vi "SearchMatch.vi"(8 "Error In":errorcluster, 11 "data_from2d3d":i32[](array[numeric])) -> (0 "Error Out":errorcluster, 1 "Elements Selected":string[][](table), 3 "data out":T2, 4 "Param Calibrazione":T1, 5 "List ROI out":dbl[][](array[numeric]))   [LabVIEW 2023]
uses:
  control/param_calibrazione.ctl
  <vilib>/Analysis/1siggen.llb/Ramp Pattern by Samples.vi
  control/global name path.vi
  queue/Front Panel Message Queue.lvlib
  <vilib>/Analysis/NI_AALBase.lvlib
panel:
  out "Saving Parth":path
  in  "name sample":bool
  in  "concentration":bool
  in  "Load Calibration":path
  out "name":string
  in  "Save":bool
  out "XY Graph":T2(graph)
  in  "select":bool
  out "Peaks Found":string[][](table)
  in  "Search Peak":bool
  in  "width":i32=80 min=3
  in  "threshold":dbl=1500.0 format="%0.2f"
  out "Spectrum":cluster{"Channels":dbl[], "Intensity":dbl[]}[](graph)
  out "Data In":T3(graph)
  in  "load":bool
  in  "open":bool
  in  "calib":bool
  in  "Stop":bool
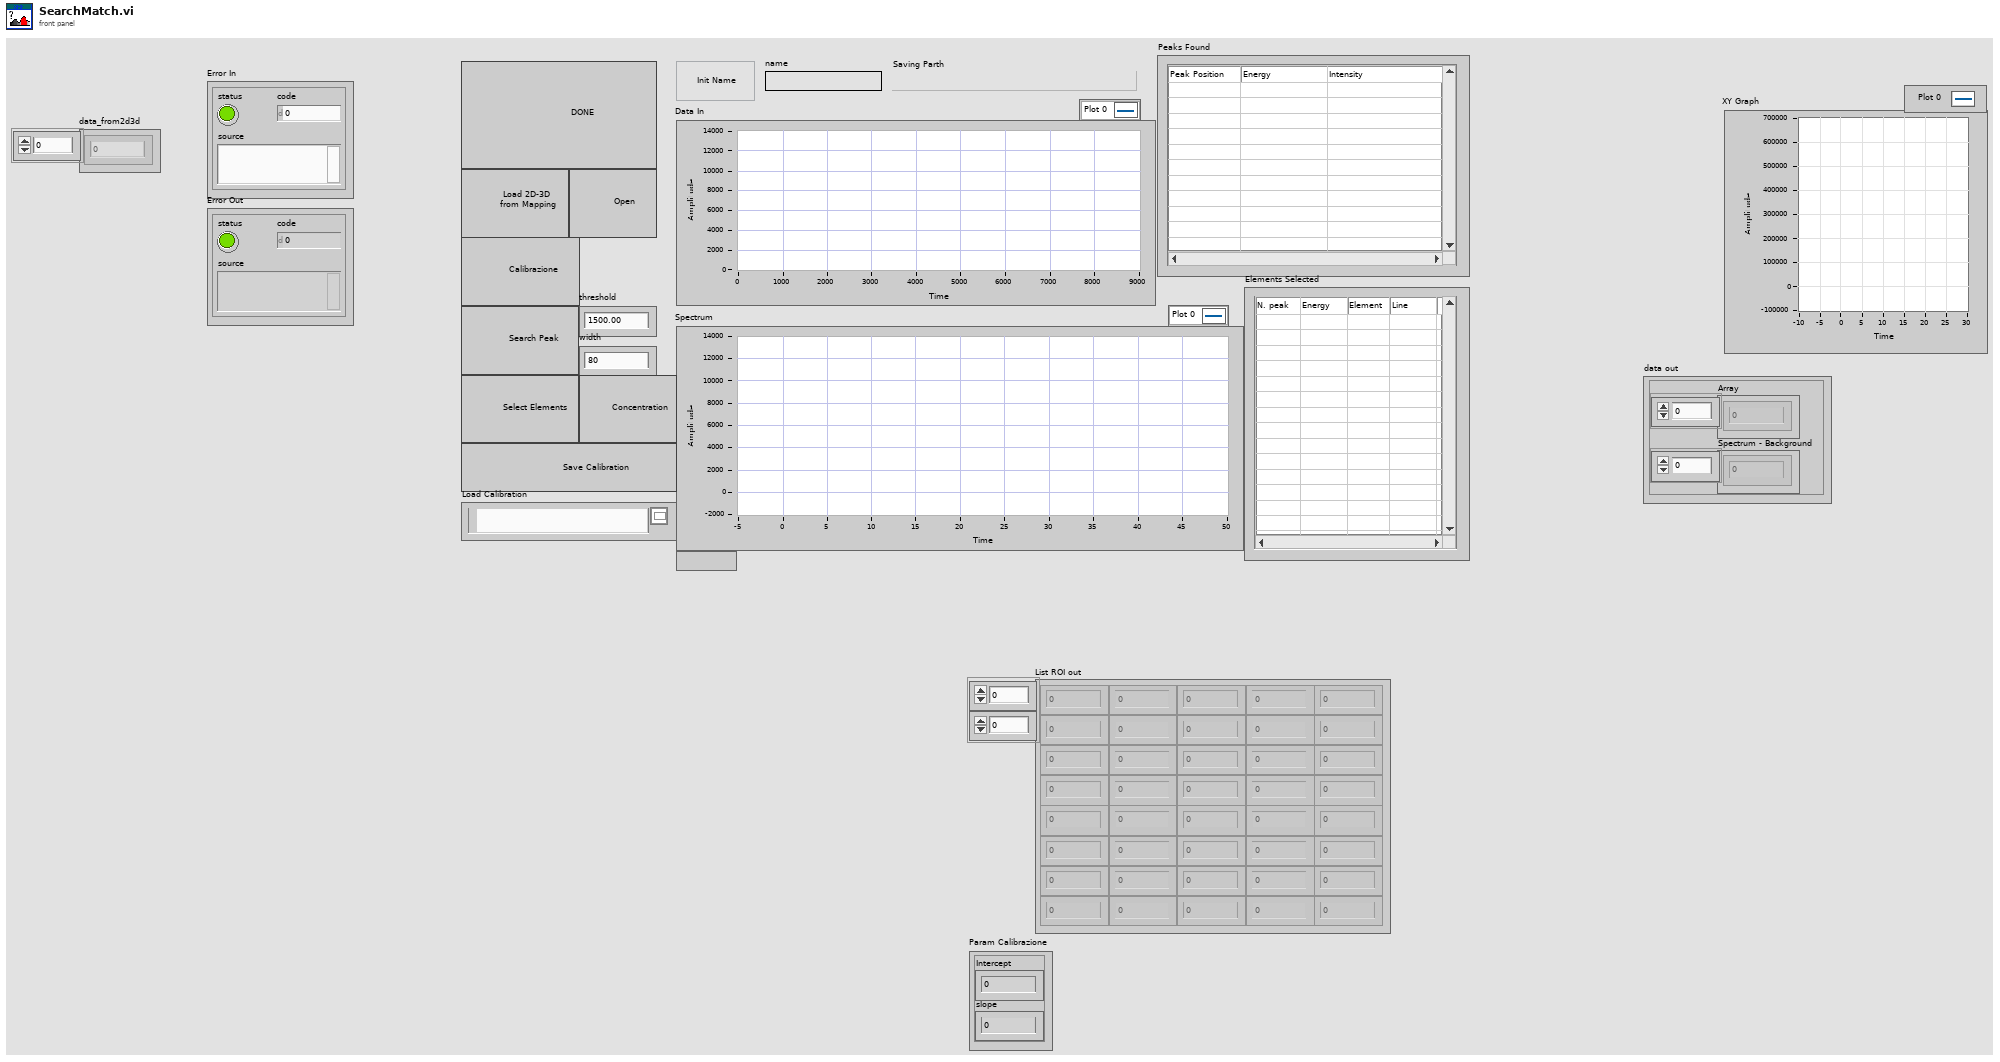
[diagram p1: front panel]
types:
  T1 = typedef "param_calibrazione.ctl" = cluster{"Intercept":dbl, "slope":dbl}
  T2 = cluster{"Array":dbl[], "Spectrum - Background":dbl[]}
  T3 = cluster{"Ramp Pattern":dbl[], "data_from2d3d":i32[]}
  T4 = typedef "Front Panel Message Queue.lvlib/Calibrazione Message Queues.ctl" = cluster{"Main":refnum<queue>, "Data":refnum<queue>}
  T5 = cluster{"Array":dbl[], "Spectrum - Background":dbl[]}[]
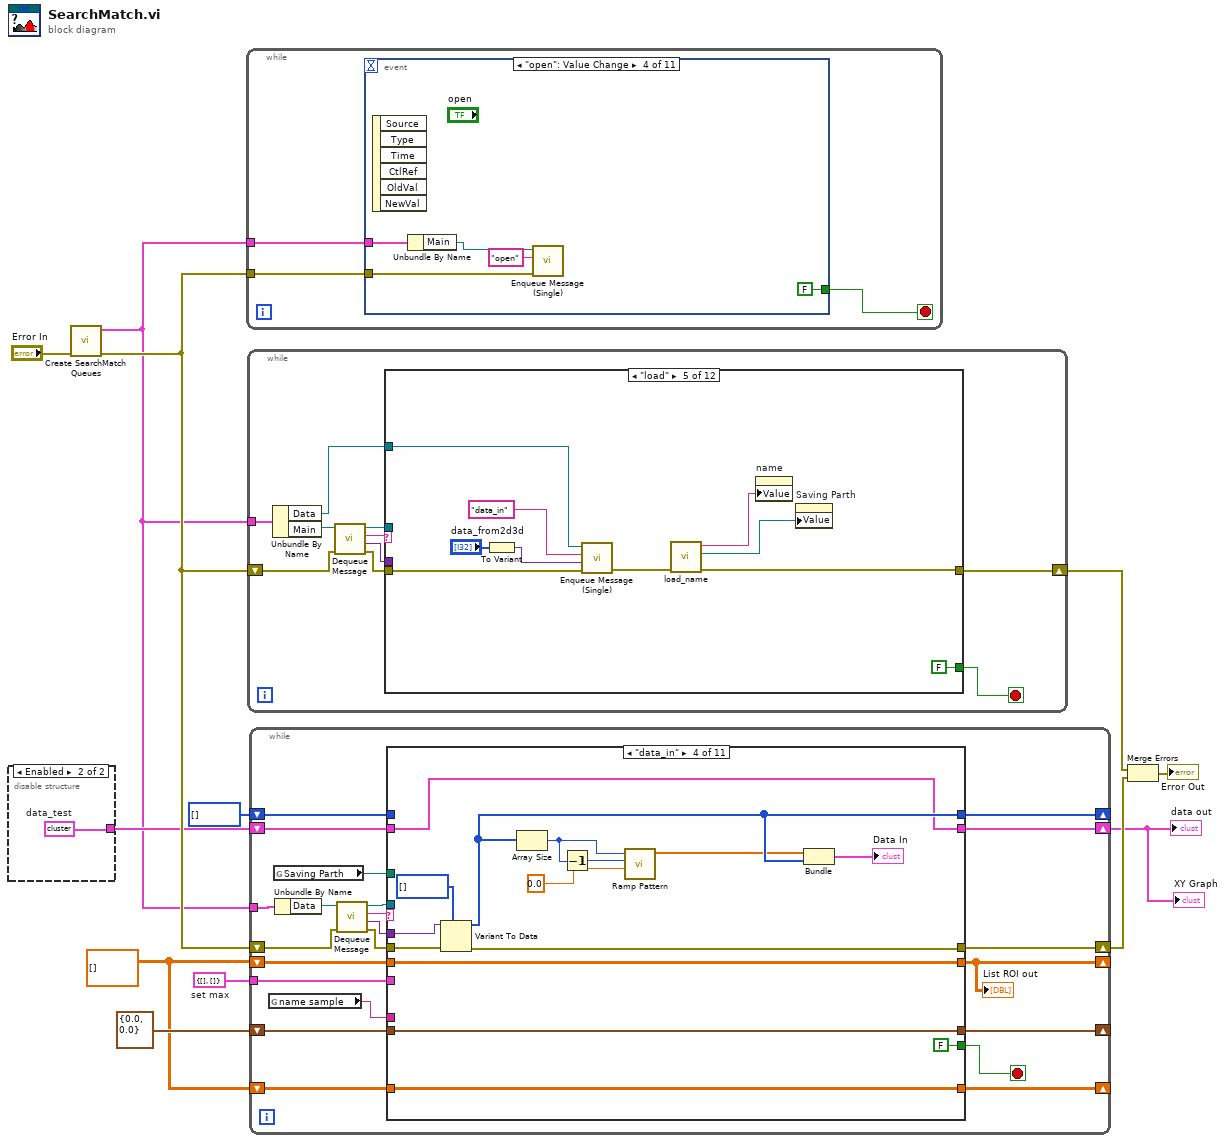
[diagram p0: block diagram]
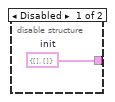
[diagram p2: hidden frame]
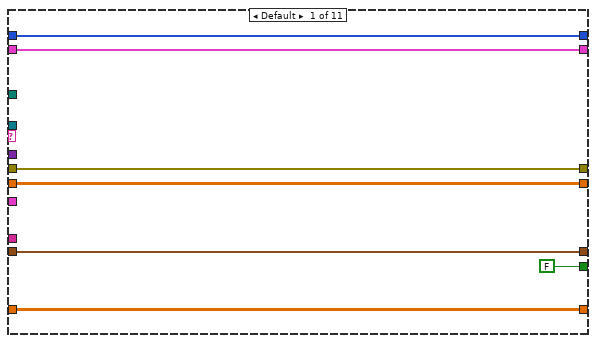
[diagram p3: hidden frame]
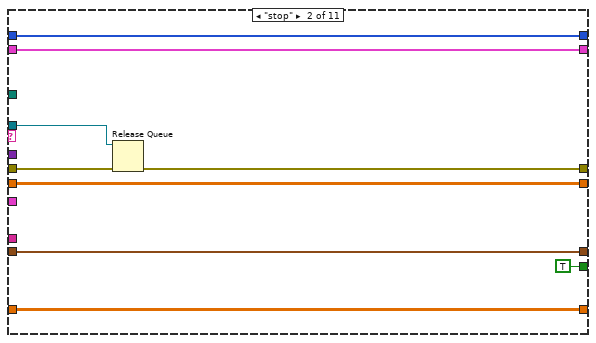
[diagram p4: hidden frame]
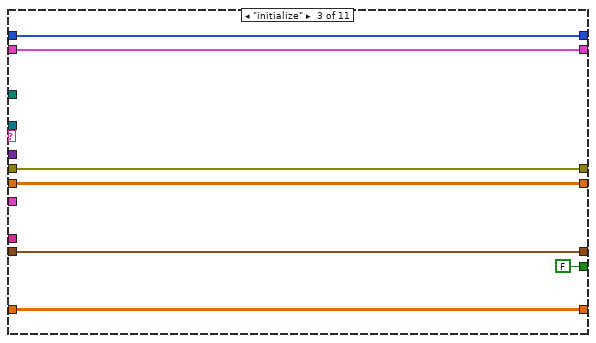
[diagram p5: hidden frame]
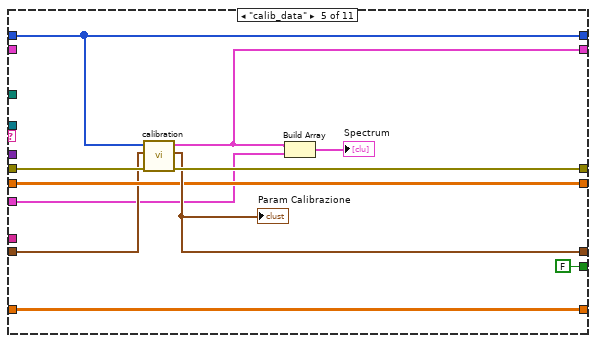
[diagram p6: hidden frame]
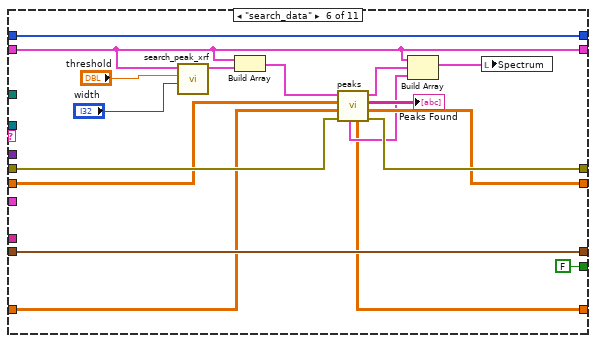
[diagram p7: hidden frame]
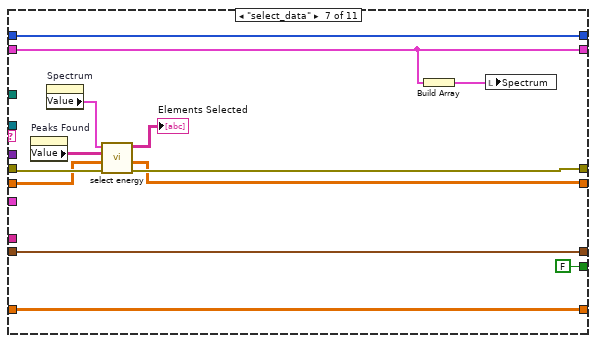
[diagram p8: hidden frame]
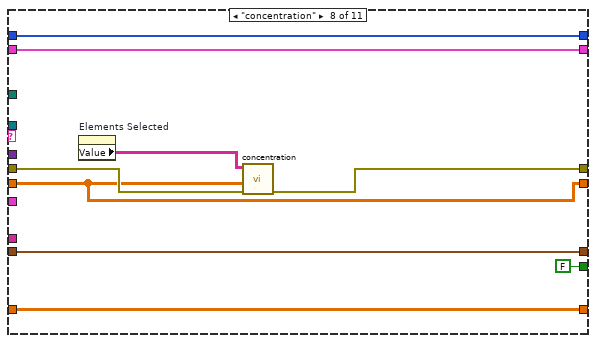
[diagram p9: hidden frame]
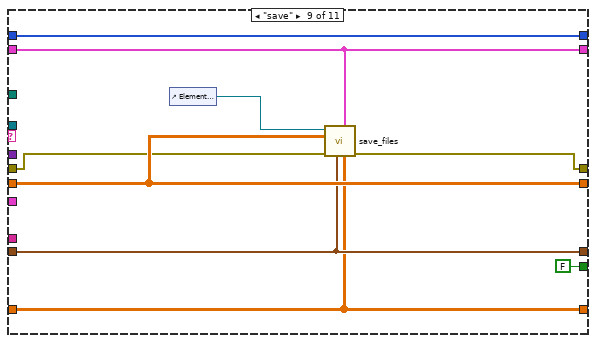
[diagram p10: hidden frame]
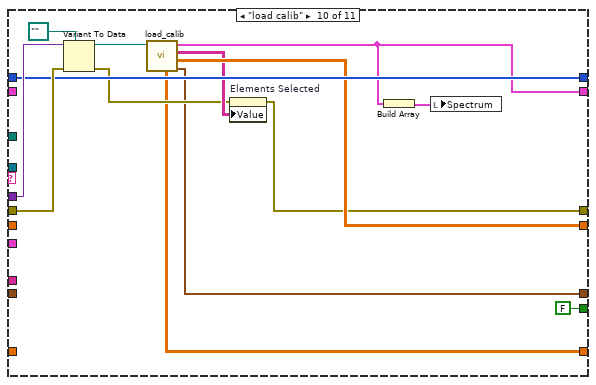
[diagram p11: hidden frame]
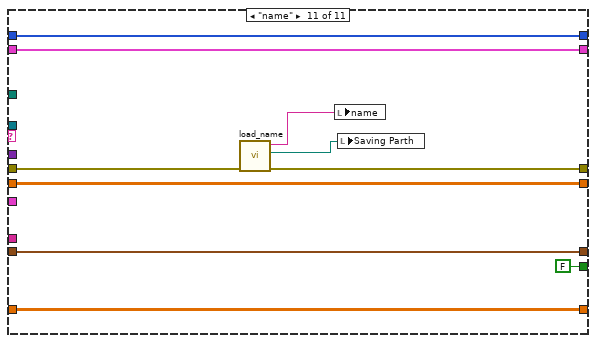
[diagram p12: hidden frame]
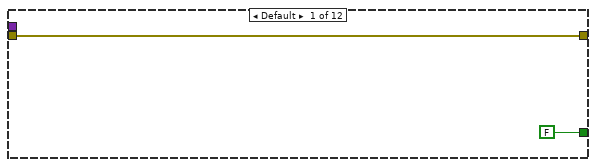
[diagram p13: hidden frame]
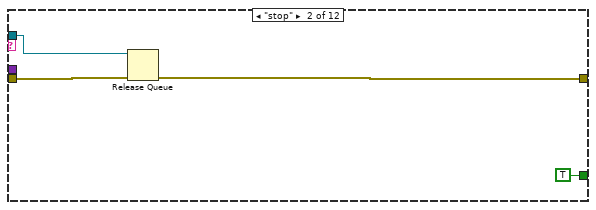
[diagram p14: hidden frame]
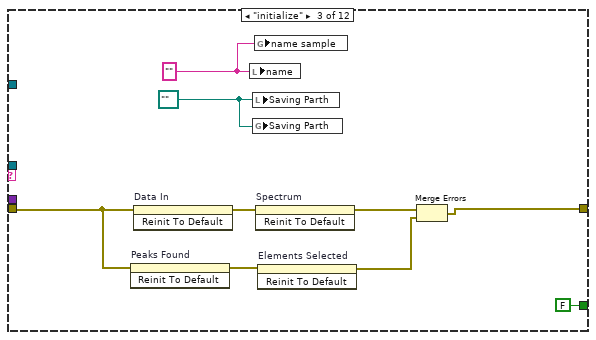
[diagram p15: hidden frame]
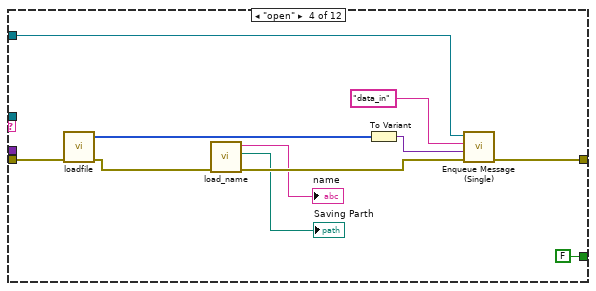
[diagram p16: hidden frame]
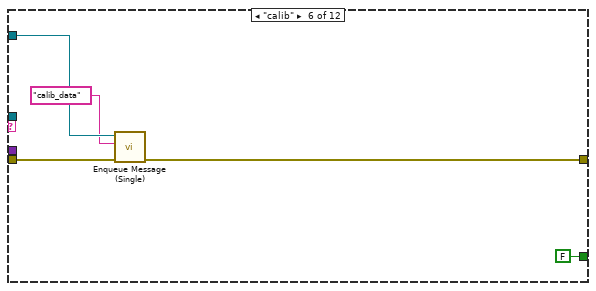
[diagram p17: hidden frame]
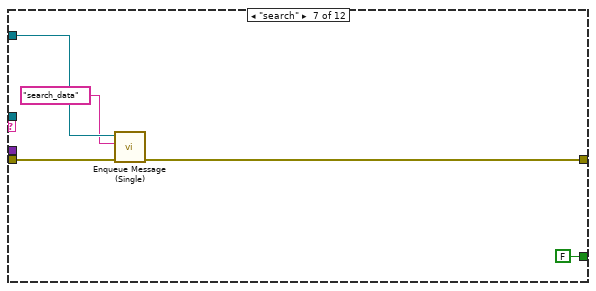
[diagram p18: hidden frame]
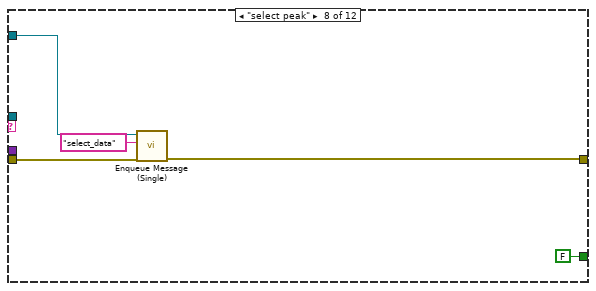
[diagram p19: hidden frame]
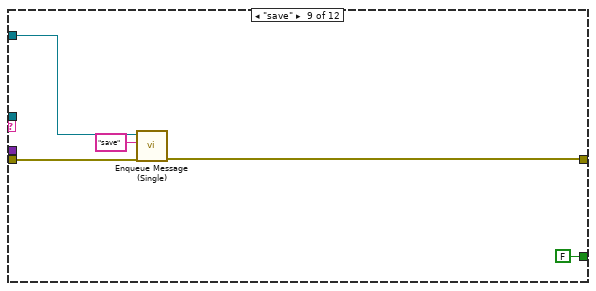
[diagram p20: hidden frame]
diagram:
  w1 = dbl[][] [] ("List ROI")
  w5 = cluster{"Channels":dbl[], "Intensity":dbl[]} {"Channels"=[], "Intensity"=[]}  # set max
  n1 = disable-structure shown="Enabled" {
    disable-tunnel: [w13 w14] -> w6
    frame Disabled {
      w13 = T2 {"Array"=[], "Spectrum - Background"=[]}  # init
    }
    frame Enabled {
      w14 = T2 {"Array"=array[8192 elements], "Spectrum - Background"=array[8192 elements]}  # data_test
    }
  }
  n2 = call "Create SearchMatch Queues.vi"("error in (no error)"="Error In") -> ("error out"=w9:errorcluster, "Message Queues"=w2:T4)  [unwired: 9 in]
  n3 = while {
    tunnel: w9 -> [w16]
    tunnel: w2 -> [w15]
    stop <- w17 stop-if-true
    n4 = event shown="[3] \"open\": Value Change" {
      selector: _ -> [_ _ _ _ _ _ _ _ _ _ _]
      dyn-events: _ -> [_ _ _ _ _ _ _ _ _ _ _]
      timeout: _ -> [_ _ _ _ _ _ _ _ _ _ _]
      tunnel: [FALSE TRUE FALSE FALSE FALSE FALSE FALSE FALSE FALSE FALSE FALSE] -> w17
      tunnel: w16 -> [_ w25 w30 w35 w41 w46 w49 w54 w61 w66 w72]
      tunnel: w15 -> [_ w24 w29 w34 w39 w44 w51 w56 w60 w65 w71]
      event Timeout {
        n5 = event-data() -> ()  [unwired: 1 in, 3 out]
      }
      event "Stop": Value Change {
        w22 = TRUE ("Priority Message? (F)")
        w21 = "stop" ("Message")
        n6 = event-data() -> ()  [unwired: 1 in, 6 out]
        n7 = Unbundle By Name(w24) -> ("Main"=w19:refnum<queue>, "Data"=w20:refnum<queue>)
        n8 = call "Enqueue Message (Single).vi"("Priority Message? (F)"=w22, "error in (no error)"=w25, "Message"=w21, "Message Queue"=w20) -> ("error out"=w23:errorcluster)  [unwired: 6 in, 1 out]
        n9 = call "Enqueue Message (Single).vi"("Priority Message? (F)"=w22, "error in (no error)"=w23, "Message"=w21, "Message Queue"=w19) -> ()  [unwired: 6 in, 2 out]
      }
      event "load": Value Change {
        n10 = event-data() -> ()  [unwired: 1 in, 6 out]
        n11 = Unbundle By Name(w29) -> ("Main"=w28:refnum<queue>)
        n12 = call "Enqueue Message (Single).vi"("error in (no error)"=w30, "Message"="load", "Message Queue"=w28) -> ()  [unwired: 7 in, 2 out]
      }
      event "open": Value Change {
        n13 = event-data() -> ()  [unwired: 1 in, 6 out]
        n14 = Unbundle By Name(w34) -> ("Main"=w33:refnum<queue>)
        n15 = call "Enqueue Message (Single).vi"("error in (no error)"=w35, "Message"="open", "Message Queue"=w33) -> ()  [unwired: 7 in, 2 out]
      }
      event "calib": Value Change {
        n16 = event-data() -> ()  [unwired: 1 in, 6 out]
        n17 = Unbundle By Name(w39) -> ("Main"=w38:refnum<queue>)
        n18 = call "Enqueue Message (Single).vi"("error in (no error)"=w41, "Message"="calib", "Message Queue"=w38) -> ()  [unwired: 7 in, 2 out]
      }
      event "Search Peak": Value Change {
        n19 = event-data() -> ()  [unwired: 1 in, 6 out]
        n20 = Unbundle By Name(w44) -> ("Main"=w43:refnum<queue>)
        n21 = call "Enqueue Message (Single).vi"("error in (no error)"=w46, "Message"="search", "Message Queue"=w43) -> ()  [unwired: 7 in, 2 out]
      }
      event "select": Value Change {
        n22 = event-data() -> ()  [unwired: 1 in, 6 out]
        n23 = Unbundle By Name(w51) -> ("Main"=w50:refnum<queue>)
        n24 = call "Enqueue Message (Single).vi"("error in (no error)"=w49, "Message"="select peak", "Message Queue"=w50) -> ()  [unwired: 7 in, 2 out]
      }
      event "Save": Value Change {
        n25 = event-data() -> ()  [unwired: 1 in, 6 out]
        n26 = Unbundle By Name(w56) -> ("Main"=w55:refnum<queue>)
        n27 = call "Enqueue Message (Single).vi"("error in (no error)"=w54, "Message"="save", "Message Queue"=w55) -> ()  [unwired: 7 in, 2 out]
      }
      event "Load Calibration": Value Change {
        n28 = event-data() -> ()  [unwired: 1 in, 6 out]
        n29 = To Variant(anything="Load Calibration") -> (Variant=w58:variant)
        n30 = Unbundle By Name(w60) -> ("Main"=w63:refnum<queue>)
        n31 = call "Enqueue Message (Single).vi"("error in (no error)"=w61, "Message Data"=w58, "Message"="load calib", "Message Queue"=w63) -> ()  [unwired: 6 in, 2 out]
      }
      event "name sample": Value Change {
        n32 = event-data() -> ()  [unwired: 1 in, 6 out]
        n33 = Unbundle By Name(w65) -> ("Main"=w68:refnum<queue>)
        n34 = call "Enqueue Message (Single).vi"("error in (no error)"=w66, "Message"="name", "Message Queue"=w68) -> ()  [unwired: 7 in, 2 out]
      }
      event "concentration": Value Change {
        n35 = event-data() -> ()  [unwired: 1 in, 6 out]
        n36 = Unbundle By Name(w71) -> ("Main"=w70:refnum<queue>)
        n37 = call "Enqueue Message (Single).vi"("error in (no error)"=w72, "Message"="concentration", "Message Queue"=w70) -> ()  [unwired: 7 in, 2 out]
      }
    }
  }
  n38 = while {
    shift-right: [w79] -> w10
    shift-left: w9 -> [w83]
    tunnel: w2 -> [w74]
    stop <- w81 stop-if-true
    n39 = Unbundle By Name(w74) -> ("Data"=w76:refnum<queue>, "Main"=w78:refnum<queue>)
    n40 = call "Dequeue Message.vi"("error in (no error)"=w83, "Message Queue"=w78) -> ("error out"=w80:errorcluster, "Message Data"=w75:variant, "Message"=w82:string, "dup Message Queue"=w77:refnum<queue>)  [unwired: 5 in, 1 out]
    n41 = case shown="\"load\"" w82 {
      tunnel: [FALSE TRUE FALSE FALSE FALSE FALSE FALSE FALSE FALSE FALSE FALSE FALSE] -> w81
      tunnel: w80 -> [w84 w88 w96 w108 w115 w123 w128 w134 w139 w145 w150 w154]
      tunnel: [w84 w87 w92 w103 w110 w122 w127 w132 w137 w143 w148 w152] -> w79
      tunnel: w77 -> [_ w86 _ _ _ _ _ _ _ _ _ _]
      tunnel: w76 -> [_ _ _ w107 w118 w121 w126 w133 w138 w144 w149 w153]
      tunnel: w75 -> [_ _ _ _ _ _ _ _ _ w140 _ _]
      frame Default {
      }
      frame "stop" {
        n42 = Release Queue(queue=w86, error in (no error)=w88) -> (error out=w87:errorcluster)  [unwired: 1 in, 2 out]
      }
      frame "initialize" {
        w91 = path ""
        w90 = ""
        n43 = invoke on="Peaks Found" class="Tbl (strict)" method="Reinit To Default"(error in=w96) -> (error out=w95:errorcluster)  [unwired: 2 in, 2 out]
        n44 = invoke on="Data In" class="XYGraph (strict)" method="Reinit To Default"(error in=w96) -> (error out=w97:errorcluster)  [unwired: 2 in, 2 out]
        n45 = local write "name"(w90) -> ()
        n46 = local write "Saving Parth"(w91) -> ()
        n47 = global write "global name path.vi" "Saving Parth"(w91) -> ()
        n48 = global write "global name path.vi" "name sample"(w90) -> ()
        n49 = invoke on="Spectrum" class="XYGraph (strict)" method="Reinit To Default"(error in=w97) -> (error out=w94:errorcluster)  [unwired: 2 in, 2 out]
        n50 = invoke on="Elements Selected" class="Tbl (strict)" method="Reinit To Default"(error in=w95) -> (error out=w93:errorcluster)  [unwired: 2 in, 2 out]
        n51 = Merge Errors(w94, w93) -> (w92:errorcluster)
      }
      frame "open" {
        n52 = call "loadfile.vi"("Error In"=w108) -> ("Error Out"=w102:errorcluster, "Data"=w106:i64[])  [unwired: 9 in]
        n53 = call "load_name.vi"("error in"=w102) -> ("error out"=w101:errorcluster, "Saving Path Out"=→"Saving Parth":path, "Name Out"=→"name":string)  [unwired: 8 in]
        n54 = To Variant(anything=w106) -> (Variant=w105:variant)
        n55 = call "Enqueue Message (Single).vi"("error in (no error)"=w101, "Message Data"=w105, "Message"="data_in", "Message Queue"=w107) -> ("error out"=w103:errorcluster)  [unwired: 6 in, 1 out]
      }
      frame "load" {
        n56 = To Variant(anything="data_from2d3d") -> (Variant=w117:variant)
        n57 = call "Enqueue Message (Single).vi"("error in (no error)"=w115, "Message Data"=w117, "Message"="data_in", "Message Queue"=w118) -> ("error out"=w111:errorcluster)  [unwired: 6 in, 1 out]
        n58 = call "load_name.vi"("error in"=w111) -> ("error out"=w110:errorcluster, "Saving Path Out"=w113:path, "Name Out"=w112:string)  [unwired: 8 in]
        n59 = property on="name" class="Str"("Value"=w112) -> ()  [unwired: 2 in, 2 out]
        n60 = property on="Saving Parth" class="Path"("Value"=w113) -> ()  [unwired: 2 in, 2 out]
      }
      frame "calib" {
        n61 = call "Enqueue Message (Single).vi"("error in (no error)"=w123, "Message"="calib_data", "Message Queue"=w121) -> ("error out"=w122:errorcluster)  [unwired: 7 in, 1 out]
      }
      frame "search" {
        n62 = call "Enqueue Message (Single).vi"("error in (no error)"=w128, "Message"="search_data", "Message Queue"=w126) -> ("error out"=w127:errorcluster)  [unwired: 7 in, 1 out]
      }
      frame "select peak" {
        n63 = call "Enqueue Message (Single).vi"("error in (no error)"=w134, "Message"="select_data", "Message Queue"=w133) -> ("error out"=w132:errorcluster)  [unwired: 7 in, 1 out]
      }
      frame "save" {
        n64 = call "Enqueue Message (Single).vi"("error in (no error)"=w139, "Message"="save", "Message Queue"=w138) -> ("error out"=w137:errorcluster)  [unwired: 7 in, 1 out]
      }
      frame "load calib" {
        n65 = call "Enqueue Message (Single).vi"("error in (no error)"=w145, "Message Data"=w140, "Message"="load calib", "Message Queue"=w144) -> ("error out"=w143:errorcluster)  [unwired: 6 in, 1 out]
      }
      frame "name" {
        n66 = call "Enqueue Message (Single).vi"("error in (no error)"=w150, "Message"="name", "Message Queue"=w149) -> ("error out"=w148:errorcluster)  [unwired: 7 in, 1 out]
      }
      frame "concentration" {
        n67 = call "Enqueue Message (Single).vi"("error in (no error)"=w154, "Message"="concentration", "Message Queue"=w153) -> ("error out"=w152:errorcluster)  [unwired: 7 in, 1 out]
      }
    }
  }
  n68 = while {
    shift-right: [w172] -> w8
    shift-left: w9 -> [w176]
    shift-right: [w169] -> _
    shift-left: i64[] [] ("data_from2d3d") -> [w168]
    shift-right: [w167] -> w3
    shift-left: w6 -> [w166]
    tunnel: w5 -> [w165]
    shift-right: [w164] -> _
    shift-left: T1 {"Intercept"=0.0, "slope"=0.0} ("Param Calibrazione") -> [w163]
    shift-right: [w162] -> _
    shift-left: w1 -> [w161]
    tunnel: w2 -> [w160]
    shift-right: [w159] -> _
    shift-left: w1 -> [w158]
    stop <- w174 stop-if-true
    n69 = global read "global name path.vi" "name sample"() -> (w156:string)
    n70 = global read "global name path.vi" "Saving Parth"() -> (w157:path)
    n71 = Unbundle By Name(w160) -> ("Data"=w177:refnum<queue>)
    n72 = call "Dequeue Message.vi"("error in (no error)"=w176, "Message Queue"=w177) -> ("error out"=w173:errorcluster, "Message Data"=w170:variant, "Message"=w175:string, "dup Message Queue"=w171:refnum<queue>)  [unwired: 5 in, 1 out]
    n73 = case shown="\"data_in\"" w175 {
      tunnel: [FALSE TRUE FALSE FALSE FALSE FALSE FALSE FALSE FALSE FALSE FALSE] -> w174
      tunnel: w173 -> [w183 w192 w199 w215 w225 w239 w255 w263 w269 w288 w293]
      tunnel: [w183 w190 w199 w212 w224 w238 w254 w262 w272 w280 w292] -> w172
      tunnel: w171 -> [_ w191 _ _ _ _ _ _ _ _ _]
      tunnel: w170 -> [_ _ _ w214 _ _ _ _ _ w287 _]
      tunnel: [w182 w189 w198 w207 w223 w242 w256 w265 w275 w284 w298] -> w169
      tunnel: w168 -> [w182 w189 w198 _ w223 w242 w256 w265 w275 w284 w298]
      tunnel: [w181 w188 w197 w204 w219 w234 w250 w264 w273 w279 w296] -> w167
      tunnel: w166 -> [w181 w188 w197 w204 _ w234 w250 w264 w273 _ w296]
      tunnel: w165 -> [_ _ _ _ w216 _ _ _ _ _ _]
      tunnel: [w180 w187 w196 w203 w221 w232 w251 w259 w270 w277 w297] -> w164
      tunnel: w163 -> [w180 w187 w196 w203 w218 w232 w251 w259 w270 _ w297]
      tunnel: [w179 w186 w195 w202 w220 w231 w246 w261 w271 w283 w295] -> w162
      tunnel: w161 -> [w179 w186 w195 w202 w220 w227 w247 w261 w271 _ w295]
      tunnel: w156 -> [_ _ _ _ _ _ _ _ _ _ _]
      tunnel: [w178 w185 w194 w201 w217 w229 w245 w258 w267 w276 w294] -> w159
      tunnel: w158 -> [w178 w185 w194 w201 w217 w228 w245 w258 w267 _ w294]
      tunnel: w157 -> [_ _ _ _ _ _ _ _ _ _ _]
      frame Default {
      }
      frame "stop" {
        n74 = Release Queue(queue=w191, error in (no error)=w192) -> (error out=w190:errorcluster)  [unwired: 1 in, 2 out]
      }
      frame "initialize" {
      }
      frame "data_in" {
        n75 = Variant To Data(error in=w215, type=i32[] [] ("data_from2d3d"), Variant=w214) -> (data=w207:i32[], error out=w212:errorcluster)
        n76 = Array Size(array=w207) -> (size(s)=w208:i32)
        n77 = Decrement(x=w208) -> (x-1=w209:i32)
        n78 = call-poly <vilib>:"Ramp Pattern.vi"("start"=0.0, "end"=w209, "samples"=w208) -> ("Ramp Pattern"=w205:dbl[])  [unwired: 7 in, 1 out]
        n79 = Bundle("Ramp Pattern"=w205, "data_from2d3d"=w207) -> (→"Data In":T3)  [unwired: 1 in]
      }
      frame "calib_data" {
        n80 = call "calibration.vi"("error in (no error)"=w225, "Pram_calib In"=w218, "Spectrum In"=w223) -> ("Error Out"=w224:errorcluster, "Param Calibrazione"=w221:T1, "Spectrum Out"=w219:T2)  [unwired: 5 in, 1 out]
        "Param Calibrazione" <- w221
        n81 = Build Array(w219, w216) -> (→"Spectrum":cluster{"Channels":dbl[], "Intensity":dbl[]}[])
      }
      frame "search_data" {
        n82 = call "search_peak_xrf.vi"("width"="width", "threshold"="threshold", "data_test"=w234) -> ("set max"=w240:cluster{"Channels":dbl[], "Intensity":dbl[]})  [unwired: 6 in, 2 out]
        n83 = Build Array(w234, w240) -> (w237:cluster{"Channels":dbl[], "Intensity":dbl[]}[])
        n84 = call "peaks.vi"("error in"=w239, "List Parameter Fit in"=w228, "List ROI in"=w227, "Spectrum In"=w237) -> ("error out"=w238:errorcluster, "List ROI out"=w231:dbl[][], "Table"=→"Peaks Found":string[][], "Peaks Out"=w235:cluster{"Locations":dbl[], "Amplitudes":dbl[]}, "List Parameter Fit Out"=w229:dbl[][], "Spectrum Fitted"=w230:cluster{"Array":dbl[], "Array":dbl[]})  [unwired: 2 in]
        n85 = Build Array(w234, w235, w230) -> (w233:cluster{"Array":dbl[], "Array":dbl[]}[])
        n86 = local write "Spectrum"(w233) -> ()
      }
      frame "select_data" {
        n87 = property on="Peaks Found" class="Tbl (strict)"() -> ("Value"=w253:string[][])  [unwired: 2 in, 2 out]
        n88 = property on="Spectrum" class="XYGraph (strict)"() -> ("Value"=w249:cluster{"Channels":dbl[], "Intensity":dbl[]}[])  [unwired: 2 in, 2 out]
        n89 = call "select energy.vi"("Error In"=w255, "List ROI in"=w247, "List Peak"=w253, "Spectrum"=w249) -> ("Error Out"=w254:errorcluster, "List ROI out"=w246:dbl[][], "Elements"=→"Elements Selected":string[][])  [unwired: 4 in, 1 out]
        n90 = Build Array(w250) -> (w252:T5)
        n91 = local write "Spectrum"(w252) -> ()
      }
      frame "concentration" {
        n92 = property on="Elements Selected" class="Tbl (strict)"() -> ("Value"=w260:string[][])  [unwired: 2 in, 2 out]
        n93 = call "concentration.vi"("error in"=w263, "List ROI in"=w261, "Elements Selected"=w260) -> ("error out"=w262:errorcluster)  [unwired: 7 in, 1 out]
      }
      frame "save" {
        n94 = control-ref of="Elements Selected"() -> (w268:refnum<vi>)
        n95 = call "save_files.vi"("List Parameter Fit"=w267, "data_test"=w273, "Param Calibrazione"=w270, "error in (no error)"=w269, "List ROI"=w271, "Table in"=w268) -> ("error out"=w272:errorcluster)  [unwired: 5 in]
      }
      frame "load calib" {
        n96 = Variant To Data(error in=w288, type=path "", Variant=w287) -> (data=w285:path, error out=w281:errorcluster)
        n97 = call "load_calib.vi"("Calibrate Spectrum"=w285) -> ("Param Calib"=w277:T1, "List"=w283:dbl[][], "Table"=w282:string[][], "Spectrum Out"=w279:cluster{"all rows":dbl[], "all rows":dbl[]}, "List Parameter Fit Out"=w276:dbl[][])  [unwired: 6 in]
        n98 = property on="Elements Selected" class="Tbl (strict)"(error in=w281, "Value"=w282) -> (error out=w280:errorcluster)  [unwired: 1 in, 1 out]
        n99 = Build Array(w279) -> (w278:cluster{"all rows":dbl[], "all rows":dbl[]}[])
        n100 = local write "Spectrum"(w278) -> ()
      }
      frame "name" {
        n101 = call "load_name.vi"("error in"=w293) -> ("error out"=w292:errorcluster, "Saving Path Out"=w290:path, "Name Out"=w291:string)  [unwired: 8 in]
        n102 = local write "name"(w291) -> ()
        n103 = local write "Saving Parth"(w290) -> ()
      }
    }
    "List ROI out" <- w162
  }
  "data out" <- w3
  "XY Graph" <- w3
  n104 = Merge Errors(w10, w8) -> (→"Error Out":errorcluster)
